vi "PicoScopeVoltsToAdc.vi"(0 "Max_adc":i16=32767, 1 "Units":dbl, 2 "Range Index":u32) -> (3 "ADC count":i16)   [LabVIEW 2024]
uses:
  ProbeInputRangesScaling.ctl
panel:
  in  "ProbeInputRangesScaling":T1={"Units"=["V", "V", "V", "V", "V", "V", "V", "V", "V", "V", "V", "V", "V", "V", "V", "V", "V", "V", "V", "V", "V", "V", "V", "A", "A", "A", "A", "A", "A", "A", "A", "A", "A", "A", "A", "A", "A", "A", "A", "A", "A", "A", "A", "A", "A", "A", "A", "A", "A", "A", "A", "A", "V", "V", "V", "V", "V", "V", "V", "V", "V", "V", "V", "V", "A", "A", "A", "A", "A", "A", "A", "A", "A", "A", "A", "A", "A", "A", "Ohm", "Ohm", "Ohm", "Ohm", "Ohm", "Ohm", "V", "V", "V", "V", "V", "V", "V", "V", "V", "V", "V", "C", "PASCALS", "PASCALS", "PASCALS", "PASCALS", "PASCALS", "PASCALS", "NA"], "Enum Text"=["10mV", "20mV", "50mV", "100mV", "200mV", "500mV", "1V", "2V", "5V", "10V", "20V", "50V", "100V", "200V", "1KV_2_5V", "1KV_5V", "1KV_12_5V", "1KV_25V", "1KV_50V", "1KV_125V", "1KV_250V", "1KV_500V", "1KV_1000V", "CURRENT_CLAMP_200A_2kA_1A", "CURRENT_CLAMP_200A_2kA_2A", "CURRENT_CLAMP_200A_2kA_5A", "CURRENT_CLAMP_200A_2kA_10A", "CURRENT_CLAMP_200A_2kA_20A", "CURRENT_CLAMP_200A_2kA_50A", "CURRENT_CLAMP_200A_2kA_100A", "CURRENT_CLAMP_200A_2kA_200A", "CURRENT_CLAMP_200A_2kA_500A", "CURRENT_CLAMP_200A_2kA_1000A", "CURRENT_CLAMP_200A_2kA_2000A", "CURRENT_CLAMP_40A_100mA", "CURRENT_CLAMP_40A_200mA", "CURRENT_CLAMP_40A_500mA", "CURRENT_CLAMP_40A_1A", "CURRENT_CLAMP_40A_2A", "CURRENT_CLAMP_40A_5A", "CURRENT_CLAMP_40A_10A", "CURRENT_CLAMP_40A_20A", "CURRENT_CLAMP_40A_40A", "CURRENT_CLAMP_2000ARMS_10A", "CURRENT_CLAMP_2000ARMS_20A", "CURRENT_CLAMP_2000ARMS_50A", "CURRENT_CLAMP_2000ARMS_100A", "CURRENT_CLAMP_2000ARMS_200A", "CURRENT_CLAMP_2000ARMS_500A", "CURRENT_CLAMP_2000ARMS_1000A", "CURRENT_CLAMP_2000ARMS_2000A", "CURRENT_CLAMP_2000ARMS_5000A", "x10_Probe_100mV", "x10_Probe_200mV", "x10_Probe_500mV", "x10_Probe_1V", "x10_Probe_2V", "x10_Probe_5V", "x10_Probe_10V", "x10_Probe_20V", "x10_Probe_50V", "x10_Probe_100V", "x10_Probe_200V", "x10_Probe_500V", "CURRENT_CLAMP_60A_2A", "CURRENT_CLAMP_60A_5A", "CURRENT_CLAMP_60A_10A", "CURRENT_CLAMP_60A_20A", "CURRENT_CLAMP_60A_50A", "CURRENT_CLAMP_60A_60A", "CURRENT_CLAMP_60A_V2_0_5A", "CURRENT_CLAMP_60A_V2_1A", "CURRENT_CLAMP_60A_V2_2A", "CURRENT_CLAMP_60A_V2_5A", "CURRENT_CLAMP_60A_V2_10A", "CURRENT_CLAMP_60A_V2_20A", "CURRENT_CLAMP_60A_V2_50A", "CURRENT_CLAMP_60A_V2_60A", "RESISTANCE_LEAD_NEG5_TO_20OHM", "RESISTANCE_LEAD_NEG50_TO_200OHM", "RESISTANCE_LEAD_NEG500_TO_2KOHM", "RESISTANCE_LEAD_NEG5K_TO_20KOHM", "RESISTANCE_LEAD_NEG50K_TO_LEAD_200KOHM", "RESISTANCE_LEAD_NEG500K_TO_LEAD_2MOHM", "RESISTANCE_LEAD_DIODE_TEST", "HT_NEG3_TO_5KV", "HT_NEG3_TO_10KV", "HT_NEG5_TO_20KV", "HT_NEG5_TO_50KV", "HT_NEG5_TO_100KV", "HT_NEG3_TO_5KV_INVERTED", "HT_NEG3_TO_10KV_INVERTED", "HT_NEG5_TO_20KV_INVERTED", "HT_NEG5_TO_50KV_INVERTED", "HT_NEG5_TO_100KV_INVERTED", "TEMPERATURE_NEG50_TO_150DEGC", "PRESSURE_SENSOR_-100k-150k_PASCALS", "PRESSURE_SENSOR_-100k_TO_400k_PASCALS", "PRESSURE_SENSOR_-200k_TO_800k_PASCALS", "PRESSURE_SENSOR_-400k_TO_1600k_PASCALS", "PRESSURE_SENSOR_-400k_TO_3400k_PASCALS", "PRESSURE_SENSOR_-150k_TO_1350k_PASCALS", "PICO_CONNECT_PROBE_OFF"], "Enum Values"=[0, 1, 2, 3, 4, 5, 6, 7, 8, 9, 10, 11, 12, 13, 6003, 6004, 6005, 6006, 6007, 6008, 6009, 6010, 6011, 4000, 4001, 4002, 4003, 4004, 4005, 4006, 4007, 4008, 4009, 4010, 5000, 5001, 5002, 5003, 5004, 5005, 5006, 5007, 5008, 6500, 6501, 6502, 6503, 6504, 6505, 6506, 6507, 6508, 32, 33, 34, 35, 36, 37, 38, 39, 40, 41, 42, 43, 10500, 10501, 10502, 10503, 10504, 10505, 10600, 10601, 10602, 10603, 10604, 10605, 10606, 10607, 7000, 7001, 7002, 7003, 7004, 7005, 7006, 8950, 8951, 8952, 8953, 8954, 8955, 8956, 8957, 8958, 8959, 9000, 9100, 9101, 9102, 9103, 9104, 9105, 1024], "MaxMin Values"=[[0.01, -0.01], [0.02, -0.02], [0.05, -0.05], [0.1, -0.1], [0.2, -0.2], [0.5, -0.5], [1.0, -1.0], [2.0, -2.0], [5.0, -5.0], [10.0, -10.0], [20.0, -20.0], [50.0, -50.0], [100.0, -100.0], [200.0, -200.0], [2.5, -2.5], [5.0, -5.0], [12.5, -12.5], [25.0, -25.0], [50.0, -50.0], [125.0, -125.0], [250.0, -250.0], [500.0, -500.0], [1000.0, -1000.0], [1.0, -1.0], [2.0, -2.0], [5.0, -5.0], [10.0, -10.0], [20.0, -20.0], [50.0, -50.0], [100.0, -100.0], [200.0, -200.0], [500.0, -500.0], [1000.0, -1000.0], [2000.0, -2000.0], [0.1, -0.1], [0.2, -0.2], [0.5, -0.5], [1.0, -1.0], [2.0, -2.0], [5.0, -5.0], [10.0, -10.0], [20.0, -20.0], [40.0, -40.0], [10.0, -10.0], [20.0, -20.0], [50.0, -50.0], [100.0, -100.0], [200.0, -200.0], [500.0, -500.0], [1000.0, -1000.0], [2000.0, -2000.0], [5000.0, -5000.0], [0.1, -0.1], [0.2, -0.2], [0.5, -0.5], [1.0, -1.0], [2.0, -2.0], [5.0, -5.0], [10.0, -10.0], [20.0, -20.0], [50.0, -50.0], [100.0, -100.0], [200.0, -200.0], [500.0, -500.0], [2.0, -2.0], [5.0, -5.0], [10.0, -10.0], [20.0, -20.0], [50.0, -50.0], [60.0, -60.0], [0.5, -0.5], [1.0, -1.0], [2.0, -2.0], [5.0, -5.0], [10.0, -10.0], [20.0, -20.0], [50.0, -50.0], [60.0, -60.0], [20.0, -5.0], [200.0, -200.0], [2000.0, -2000.0], [20000.0, -5000.0], [20000.0, -5000.0], [20000.0, -5000.0], [2.0, -2.0], [5000.0, -5000.0], [1000.0, -1000.0], [20000.0, -2000.0], [50000.0, -5000.0], [10000.0, -1000.0], [5000.0, -5000.0], [1000.0, -1000.0], [20000.0, -2000.0], [50000.0, -5000.0], [10000.0, -1000.0], [150.0, -50.0], [100.0, -100.0], [100.0, -100.0], [100.0, -100.0], [100.0, -100.0], [100.0, -100.0], [100.0, -100.0], [0.0, 0.0]]}
  out "Unit":string
  out "Probe Range":string
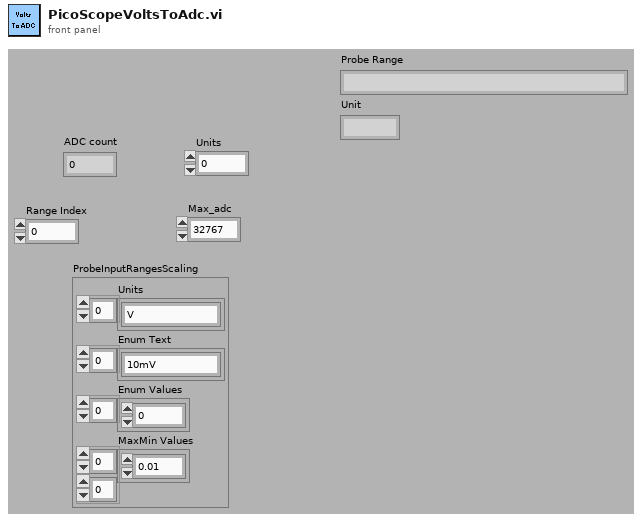
[diagram p1: front panel]
types:
  T1 = typedef "ProbeInputRangesScaling.ctl" = cluster{"Units":string[], "Enum Text":string[], "Enum Values":u32[], "MaxMin Values":dbl[][]}
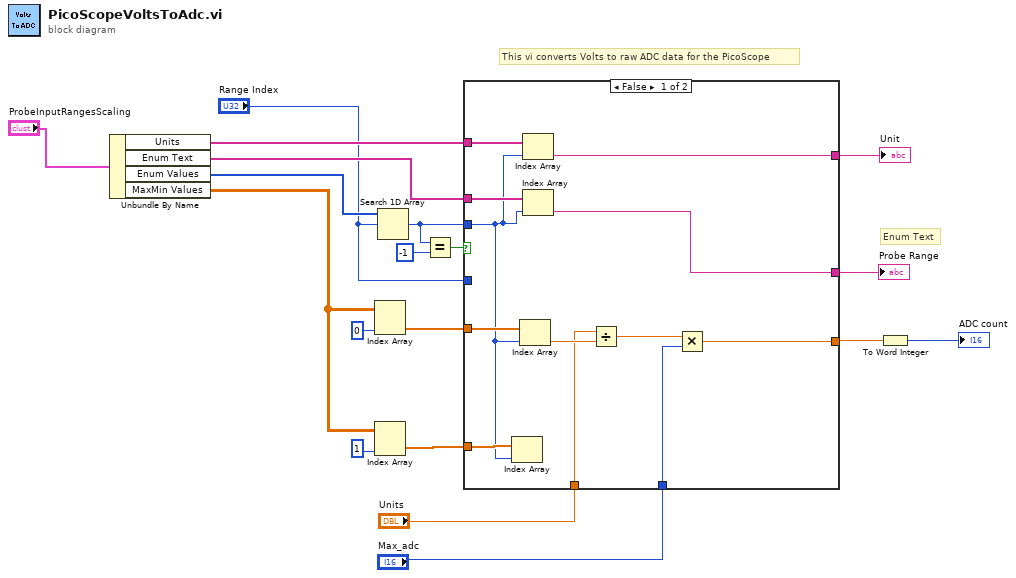
[diagram p0: block diagram]
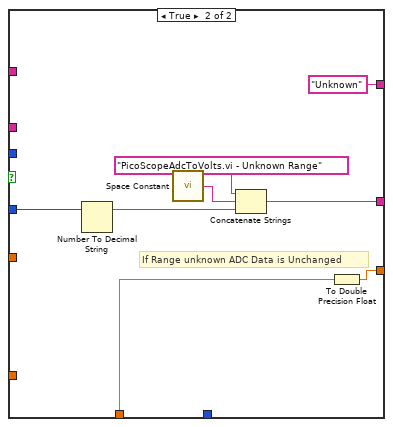
[diagram p2: hidden frame]
diagram:
  # "Enum Text"
  # "This vi converts Volts to raw ADC data for the PicoScope"
  n1 = Unbundle By Name("ProbeInputRangesScaling") -> ("Units"=w5:string[], "Enum Text"=w4:string[], "Enum Values"=w3:u32[], "MaxMin Values"=w2:dbl[][])
  n2 = Index Array(array=w2, index (col)=0 ("index (page)")) -> (element=w15:dbl[])  [unwired: 1 in]
  n3 = Index Array(array=w2, index (col)=1 ("index (page)")) -> (element=w14:dbl[])  [unwired: 1 in]
  n4 = Search 1D Array(1D array=w3, element="Range Index") -> (index of element=w17:i32)  [unwired: 1 in]
  n5 = Equal?(x=w17, y=-1) -> (x = y?=w18:bool)
  n6 = case shown="False" w18 {
    tunnel: w17 -> [w25 _]
    tunnel: "Max_adc" -> [w23 _]
    tunnel: "Units" -> [w20 w32]
    tunnel: [w22 w33] -> w7
    tunnel: "Range Index" -> [_ w39]
    tunnel: w15 -> [w31 _]
    tunnel: w14 -> [w30 _]
    tunnel: w4 -> [w29 _]
    tunnel: [w28 w38] -> w11
    tunnel: w5 -> [w27 _]
    tunnel: [w26 "Unknown" ("String")] -> w10
    frame False {
      n7 = Index Array(array=w30, index=w25) -> ()  [unwired: 1 out]
      n8 = Index Array(array=w31, index=w25) -> (element=w21:dbl)
      n9 = Index Array(array=w27, index=w25) -> (element=w26:string)
      n10 = Index Array(array=w29, index=w25) -> (element=w28:string)
      n11 = Divide(x=w20, y=w21) -> (x/y=w24:dbl)
      n12 = Multiply(x=w24, y=w23) -> (x*y=w22:dbl)
    }
    frame True {
      # "If Range unknown ADC Data is Unchanged"
      n13 = Number To Decimal String(number=w39) -> (decimal integer string=w36:string)  [unwired: 1 in]
      n14 = call <vilib>:"Space Constant.vi"() -> ("String"=w37:string)
      n15 = Concatenate Strings("PicoScopeAdcToVolts.vi - Unknown Range" ("String"), w37, w36) -> (w38:string)
      n16 = To Double Precision Float(number=w32) -> (double precision float=w33:dbl)
    }
  }
  "Probe Range" <- w11
  "Unit" <- w10
  n17 = To Word Integer(number=w7) -> (16bit integer=→"ADC count":i16)
